vi "GetCaptorData.vi"(6 "Graph in":cluster{dbl[], dbl[]}, 8 "error in":errorcluster, 9 "Length":i32=250, 11 "ON":bool) -> (0 "error out":errorcluster, 2 "Values":cluster{dbl[], dbl[]})   [LabVIEW 2013]
uses:
  GlobalVariables/HardwarePresent.vi
  GlobalVariables/CurrentPressure.vi
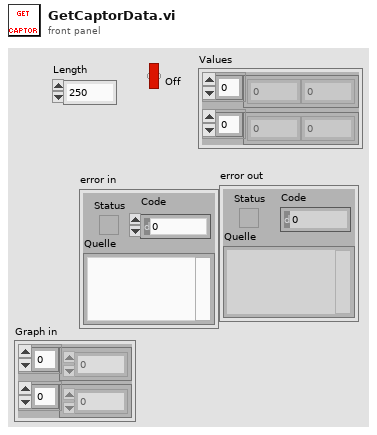
[diagram p1: front panel]
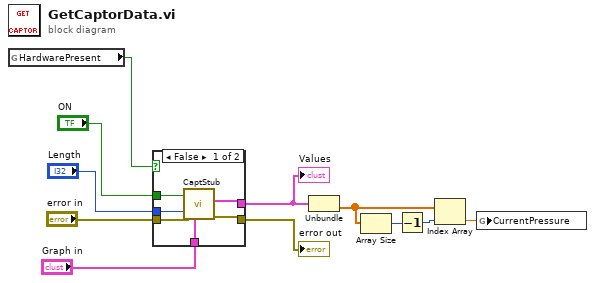
[diagram p0: block diagram]
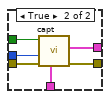
[diagram p2: hidden frame]
diagram:
  n1 = global read "HardwarePresent.vi" "HardwarePresent"() -> (w1:bool)
  n2 = case shown="False" w1 {
    tunnel: "Graph in" -> [w15 w23]
    tunnel: "error in" -> [w14 w22]
    tunnel: [w17 w21] -> w5
    tunnel: [w16 w20] -> w4
    tunnel: "Length" -> [w13 w19]
    tunnel: "ON" -> [w12 w18]
    frame False {
      n3 = call "CaptStub.vi"("Graph in"=w15, "error in"=w14, "Length"=w13, "ON"=w12) -> ("error out"=w17:errorcluster, "Values"=w16:cluster{dbl[], dbl[]})  [unwired: 6 in]
    }
    frame True {
      n4 = call "capt.vi"("Graph in"=w23, "error in"=w22, "Length"=w19, "ON"=w18) -> ("error out"=w21:errorcluster, "Values"=w20:cluster{dbl[], dbl[]})  [unwired: 6 in]
    }
  }
  "error out" <- w5
  "Values" <- w4
  n5 = Unbundle(w4) -> (w11:dbl[])  [unwired: 1 out]
  n6 = Array Size(array=w11) -> (size(s)=w10:i32)
  n7 = Decrement(x=w10) -> (x-1=w9:i32)
  n8 = Index Array(array=w11, index=w9) -> (element=w8:dbl)
  n9 = global write "CurrentPressure.vi" "CurrentPressure"(w8) -> ()
